vi "CreateHardwareDataStructures.vi"(8 "Error In":errorcluster) -> (0 "Error Out":errorcluster, 3 "Hardware Data Structures":T1)   [LabVIEW 2012]
uses:
  HardwareDataStructures.ctl
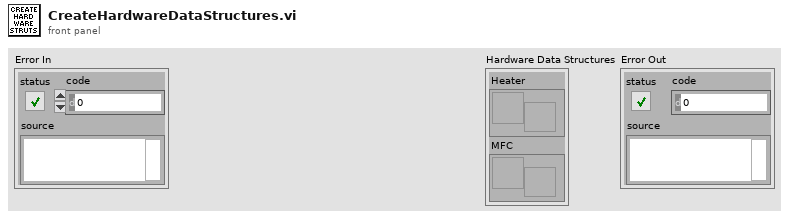
[diagram p1: front panel]
types:
  T1 = typedef "HardwareDataStructures.ctl" = cluster{"Heater":refnum<notifier>, "MFC":refnum<notifier>}
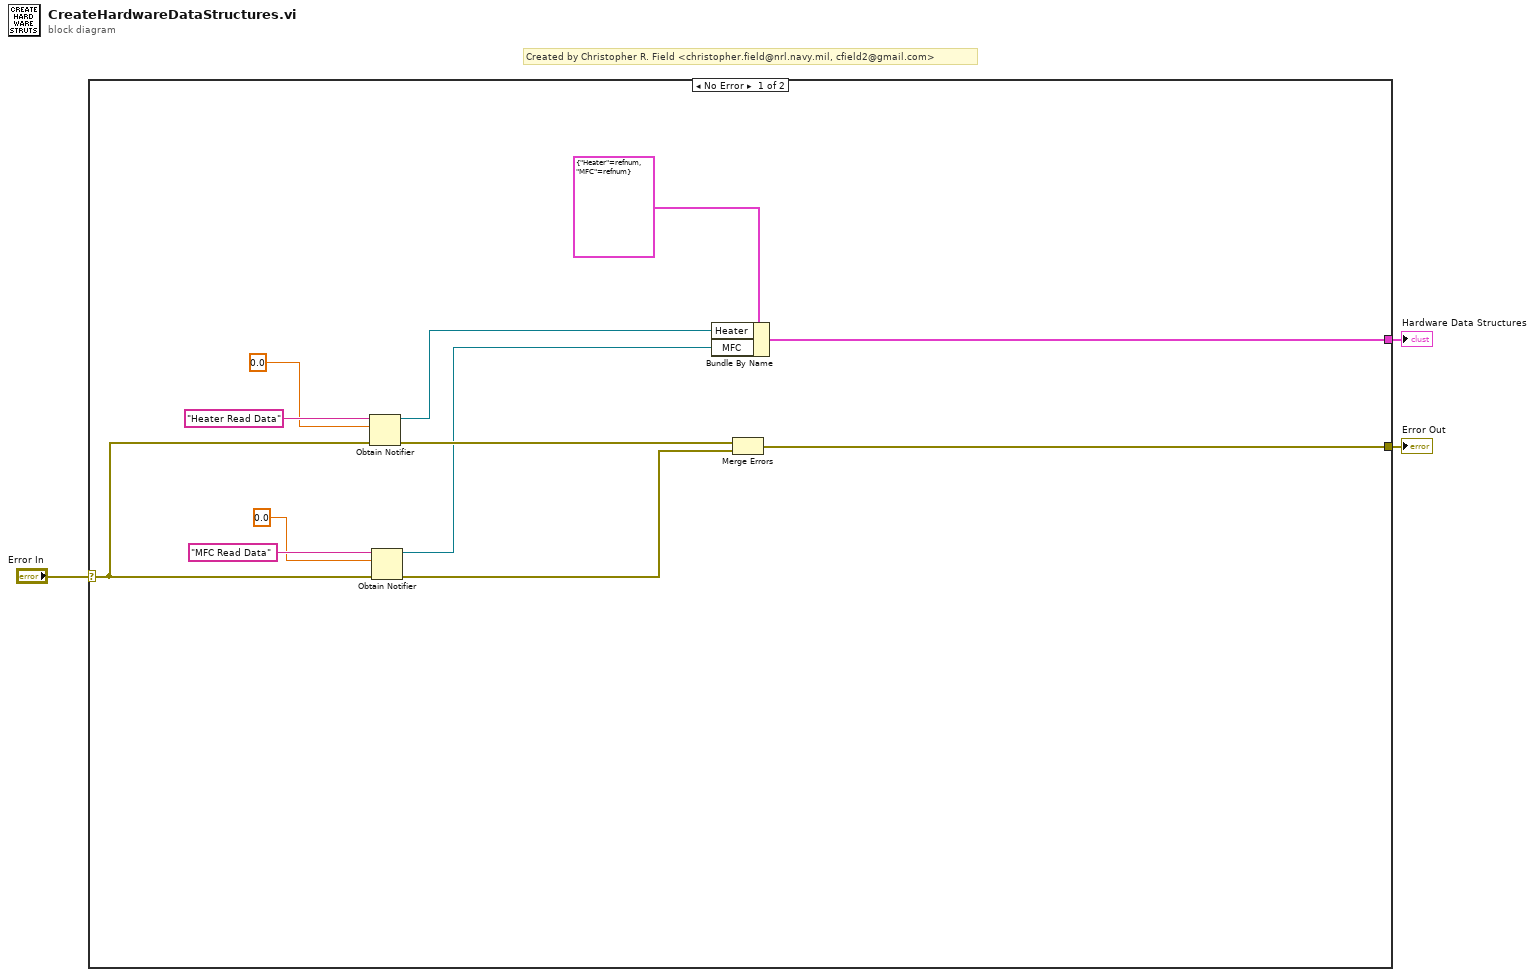
[diagram p0: block diagram]
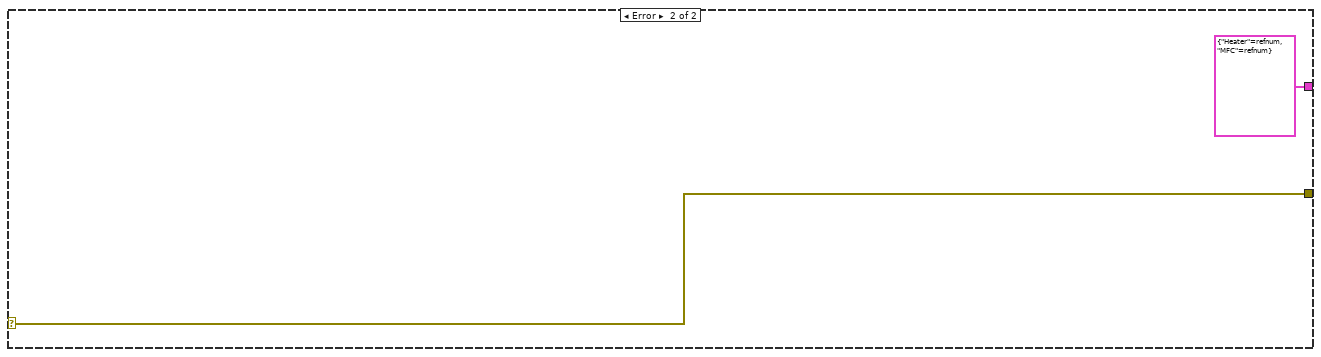
[diagram p2: hidden frame]
diagram:
  # "Created by Christopher R. Field <christopher.field@nrl.navy.mil, cfield2@gmail.com>"
  n1 = case shown="No Error" "Error In" {
    selector: "Error In" -> [w12 w17]
    tunnel: [w9 w17] -> w1
    tunnel: [w8 T1 {"Heater"=refnum, "MFC"=refnum} ("Hardware Data Structures")] -> w2
    frame No Error {
      n2 = Obtain Notifier(name (unnamed)="Heater Read Data", notification data type=0.0, error in (no error)=w12) -> (notifier out=w5:refnum<notifier>, error out=w11:errorcluster)  [unwired: 1 in, 1 out]
      n3 = Obtain Notifier(name (unnamed)="MFC Read Data", notification data type=0.0, error in (no error)=w12) -> (notifier out=w4:refnum<notifier>, error out=w10:errorcluster)  [unwired: 1 in, 1 out]
      n4 = Bundle By Name(cluster=T1 {"Heater"=refnum, "MFC"=refnum} ("Hardware Data Structures"), "Heater"=w5, "MFC"=w4) -> (w8:T1)
      n5 = Merge Errors(w11, w10) -> (w9:errorcluster)
    }
    frame Error {
    }
  }
  "Hardware Data Structures" <- w2
  "Error Out" <- w1
